vi "IEC - Third-octave Analysis.vi"(0 "scaled signal [EU]":dbl[](array[numeric]) format="%.2f", 1 "sampling frequency [Hz]":dbl=10000.0 format="%.2f", 2 "frequency range":T2={"low band"=enum."125 Hz", "high band"=enum."8000 Hz"}, 3 "dB On (T)":bool=TRUE, 5 "channel info":T3={"sensor sensitivity [mV/EU]"=1000.0, "engineering units"=1, "dB reference [EU]"=1.0, "custom label"="EU", "weighting filter"=0, "pregain [dB]"=0.0} {"pregain [dB]" format="%.2f"; "weighting filter" items=["Linear", "A-weighting", "B-weighting", "C-weighting", "ITU-R 468-4", "Dolby", "CCITT", "C-message"]; "dB reference [EU]" format="%^.1e"; "engineering units" items=["custom..."=0, "V"=1, "A"=21, "Pa"=2, "N"=20, "g"=3, "m/s^2"=4, "m/s"=5, "m"=6, "mm/s"=12, "mm"=13, "microns/s"=14, "microns"=15, "in/s^2"=7, "in/s"=8, "in"=9, "mils/s"=10, "mils"=11, "rad/s^2"=16, "rad/s"=17, "rad"=18, "strain"=19]; "sensor sensitivity [mV/EU]" format="%.2f"}, 6 "averaging type":T7(ring)=enum."Exponential", 7 "filter init/cont (init:F)":bool, 8 "averaging parameters":T1={"linear mode"=enum."start averaging once settled", "exponential mode"=enum."Fast", "time constant [ms]"=125.0, "confidence [dB]"=1.0, "peak mode"=enum."start peak detection once settled"} {"confidence [dB]" min=0.01 max=10.0 format="%.2f"; "time constant [ms]" min=0.0 format="%.2f"}, 9 "reset averaging (F)":bool) -> (12 "nominal frequencies (string)":string[](array[string]), 13 "bandedge frequencies [Hz]":T6(array[cluster]) {"midband" format="%.2f"; "f high" format="%.2f"; "f low" format="%.2f"}, 14 "band power [dB EU]":dbl[](array[numeric]) format="%.2f", 15 "unit label":string, 16 "nominal frequencies [Hz]":dbl[](array[numeric]) format="%.2f", 17 "total band power [dB EU]":dbl format="%.2f", 18 "settled?":bool, 19 "error":bool)   [LabVIEW 2017]
doc: "Performs a third-octave analysis on the input signal. The third-octave filters are designed as third-octave-band filters, class 1, IEC 1260:1995. To meet this standard, the sampling frequency must be at least 2.5 times the highest midband frequency.\nAvailable averaging types are Linear, Exponential (default), Equal confidence, and Peak. Based on the selected averaging type, this VI uses the additional settings in averaging parameters.\nThis VI returns the power in each third-octave band and the total band power, both expressed in decibels. The total band power is defined as the sum of the individual band powers.\nTo ensure a continuous filtering operation call this VI the first time with filter init/cont set to FALSE and then call it with filter init/cont set to TRUE."
uses:
  <vilib>/addons/Sound and Vibration/compatibility/Controls/svl_Channel Info.ctl
  <vilib>/addons/Sound and Vibration/compatibility/Controls/svl_Engineering Units Text Ring.ctl
  <vilib>/addons/Sound and Vibration/compatibility/Controls/svl_Weighting Filter Text Ring.ctl
  <vilib>/addons/_NISVFA/_Shared subVIs/Controls/svc_Octave Standard.ctl
  <vilib>/addons/Sound and Vibration/svt_Octave/SoundVib_Octave_2014 standard.lvlib
panel:
  # "Linear"
  # "Exponential"
  # "Equal confidence"
  # "Peak"
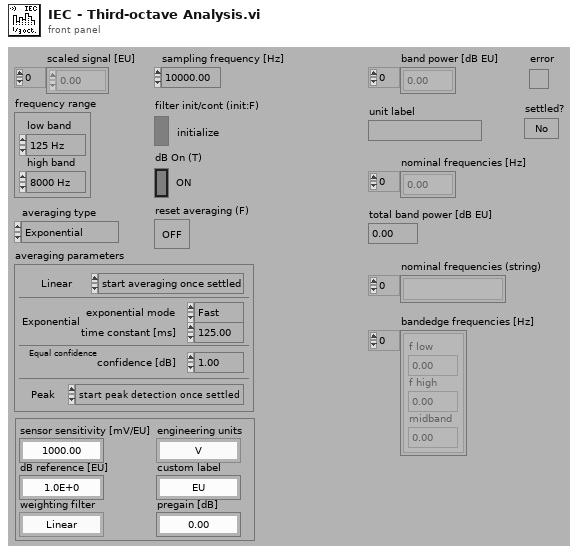
[diagram p1: front panel]
types:
  T1 = cluster{"linear mode":enum16{"start averaging once settled", "continuous averaging", "single averaging"}, "exponential mode":enum16{"Slow", "Fast", "Impulse", "Custom"}, "time constant [ms]":dbl, "confidence [dB]":dbl, "peak mode":enum16{"start peak detection once settled", "continuous peak detection", "single peak detection"}}
  T2 = cluster{"low band":enum16{"20 Hz", "25 Hz", "31.5 Hz", "40 Hz", "50 Hz", "63 Hz", "80 Hz", "100 Hz", "125 Hz", "160 Hz", "200 Hz", "250 Hz", "315 Hz", "400 Hz", "500 Hz", "630 Hz", "800 Hz", "1000 Hz", "1250 Hz", "1600 Hz", "2000 Hz", "2500 Hz", "3150 Hz", "4000 Hz", "5000 Hz", "6300 Hz", "8000 Hz", "10000 Hz", "12500 Hz", "16000 Hz", "20000 Hz"}, "high band":enum16{"20 Hz", "25 Hz", "31.5 Hz", "40 Hz", "50 Hz", "63 Hz", "80 Hz", "100 Hz", "125 Hz", "160 Hz", "200 Hz", "250 Hz", "315 Hz", "400 Hz", "500 Hz", "630 Hz", "800 Hz", "1000 Hz", "1250 Hz", "1600 Hz", "2000 Hz", "2500 Hz", "3150 Hz", "4000 Hz", "5000 Hz", "6300 Hz", "8000 Hz", "10000 Hz", "12500 Hz", "16000 Hz", "20000 Hz"}}
  T3 = typedef "svl_Channel Info.ctl" = cluster{"sensor sensitivity [mV/EU]":dbl, "engineering units":T4, "dB reference [EU]":dbl, "custom label":string, "weighting filter":T5, "pregain [dB]":dbl}
  T4 = typedef "svl_Engineering Units Text Ring.ctl" = u16
  T5 = typedef "svl_Weighting Filter Text Ring.ctl" = u16
  T6 = cluster{"f low":dbl, "f high":dbl, "midband":dbl}[]
  T7 = enum16{"Linear", "Exponential", "Equal confidence", "Peak"}
  T8 = typedef "svc_Octave Standard.ctl" = enum16{"ANSI S1.11", "IEC 61260"}
  T9 = enum16{"1 octave", "1/3 octave", "1/6 octave", "1/12 octave", "1/24 octave"}
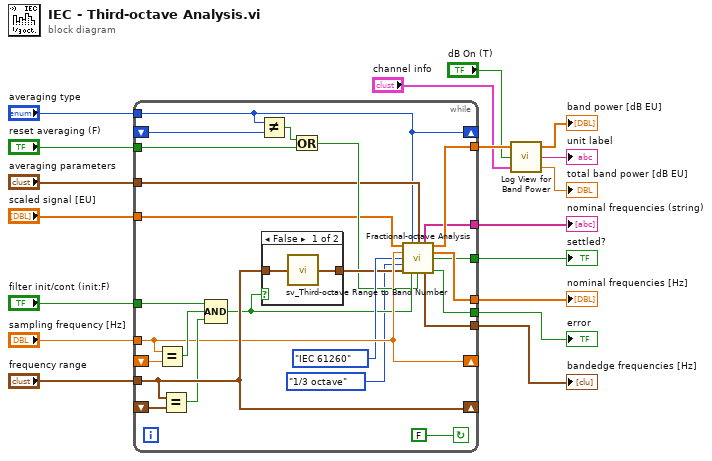
[diagram p0: block diagram]
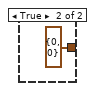
[diagram p2: hidden frame]
diagram:
  n1 = while {
    tunnel: "scaled signal [EU]" -> [w20]
    tunnel: "averaging parameters" -> [w24]
    tunnel: "reset averaging (F)" -> [w25]
    tunnel: "averaging type" -> [w23]
    shift-left: _ -> [w22]
    shift-right: [w23] -> _
    tunnel: [w28] -> w12
    tunnel: [w30] -> w13
    tunnel: [w29] -> w14
    tunnel: [w31] -> w15
    tunnel: [w32] -> w16
    tunnel: [w33] -> w11
    tunnel: "sampling frequency [Hz]" -> [w37]
    shift-left: _ -> [w41]
    shift-right: [w37] -> _
    tunnel: "frequency range" -> [w42]
    shift-left: _ -> [w43]
    shift-right: [w42] -> _
    tunnel: "filter init/cont (init:F)" -> [w40]
    stop <- FALSE continue-if-true
    n2 = Equal?(x=w37, y=w41) -> (x = y?=w38:bool)
    n3 = Equal?(x=w42, y=w43) -> (x = y?=w39:bool)
    n4 = Compound Arithmetic op=AND(w40, w38, w39) -> (w35:bool)
    n5 = Not Equal?(x=w23, y=w22) -> (x != y?=w27:bool)
    n6 = case shown="False" w35 {
      tunnel: w42 -> [w44 _]
      tunnel: [w45 cluster{"Low band":i32, "High band":i32} {"Low band"=0, "High band"=0} ("Band number")] -> w34
      frame False {
        n7 = call <vilib>:"sv_Third-octave Range to Band Number.vi"("frequency range"=w44) -> ("band number"=w45:cluster{"low band":i32, "high band":i32})
      }
      frame True {
      }
    }
    n8 = Or(x=w27, y=w25) -> (x .or. y?=w26:bool)
    n9 = call <vilib>:"Fractional-octave Analysis.vi"("scaled signal [EU]"=w20, "averaging type"=w23, "averaging parameters"=w24, "sampling frequency [Hz]"=w37, "standard"=svc_Octave_Standard."IEC 61260" ("Standard"), "bandwidth"=T9."1/3 octave" ("Bandwidth"), "band number"=w34, "filter init/cont (init:F)"=w35, "reset averaging (F)"=w26) -> ("nominal frequencies (string)"=w31:string[], "band power [EU^2 rms]"=w33:dbl[], "nominal frequencies [Hz]"=w32:dbl[], "settled?"=w29:bool, "bandedge frequencies [Hz]"=w30:T6, "error"=w28:bool)  [unwired: 1 in]
  }
  "error" <- w12
  "nominal frequencies [Hz]" <- w16
  "settled?" <- w14
  "nominal frequencies (string)" <- w15
  "bandedge frequencies [Hz]" <- w13
  n10 = call <vilib>:"Log View for Band Power.vi"("channel info"="channel info", "dB On (T)"="dB On (T)", "band power [EU^2 rms]"=w11) -> ("total band power [dB EU]"=→"total band power [dB EU]":dbl, "unit label"=→"unit label":string, "log view band power [dB EU]"=→"band power [dB EU]":dbl[])
